vi "seat leak test.vi"(7 "LabVIEW Web Service Request":refnum<class "Web Request.lvclass">, 10 "testPressure":dbl, 11 "time":dbl) -> ()   [LabVIEW 2015]
uses:
  <vilib>/wsapi/Web Request.lvclass
  <vilib>/Waveform/WDTOps.llb/WDT Append Waveforms DBL.vi
panel:
  out "value":string
  in  "Start timer":bool
  out "Final Pressure":dbl
  out "data":waveform(dbl)[](graph)
  out "timer":dbl
  in  "Stop timer":bool
  in  "Stop (Pressure Reading)":bool
  out "Starting Pressure":dbl format="%#_2g"
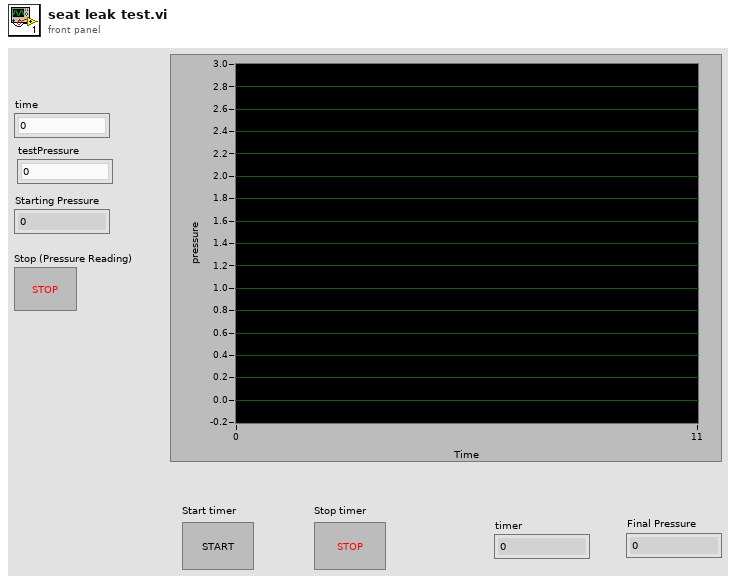
[diagram p1: front panel]
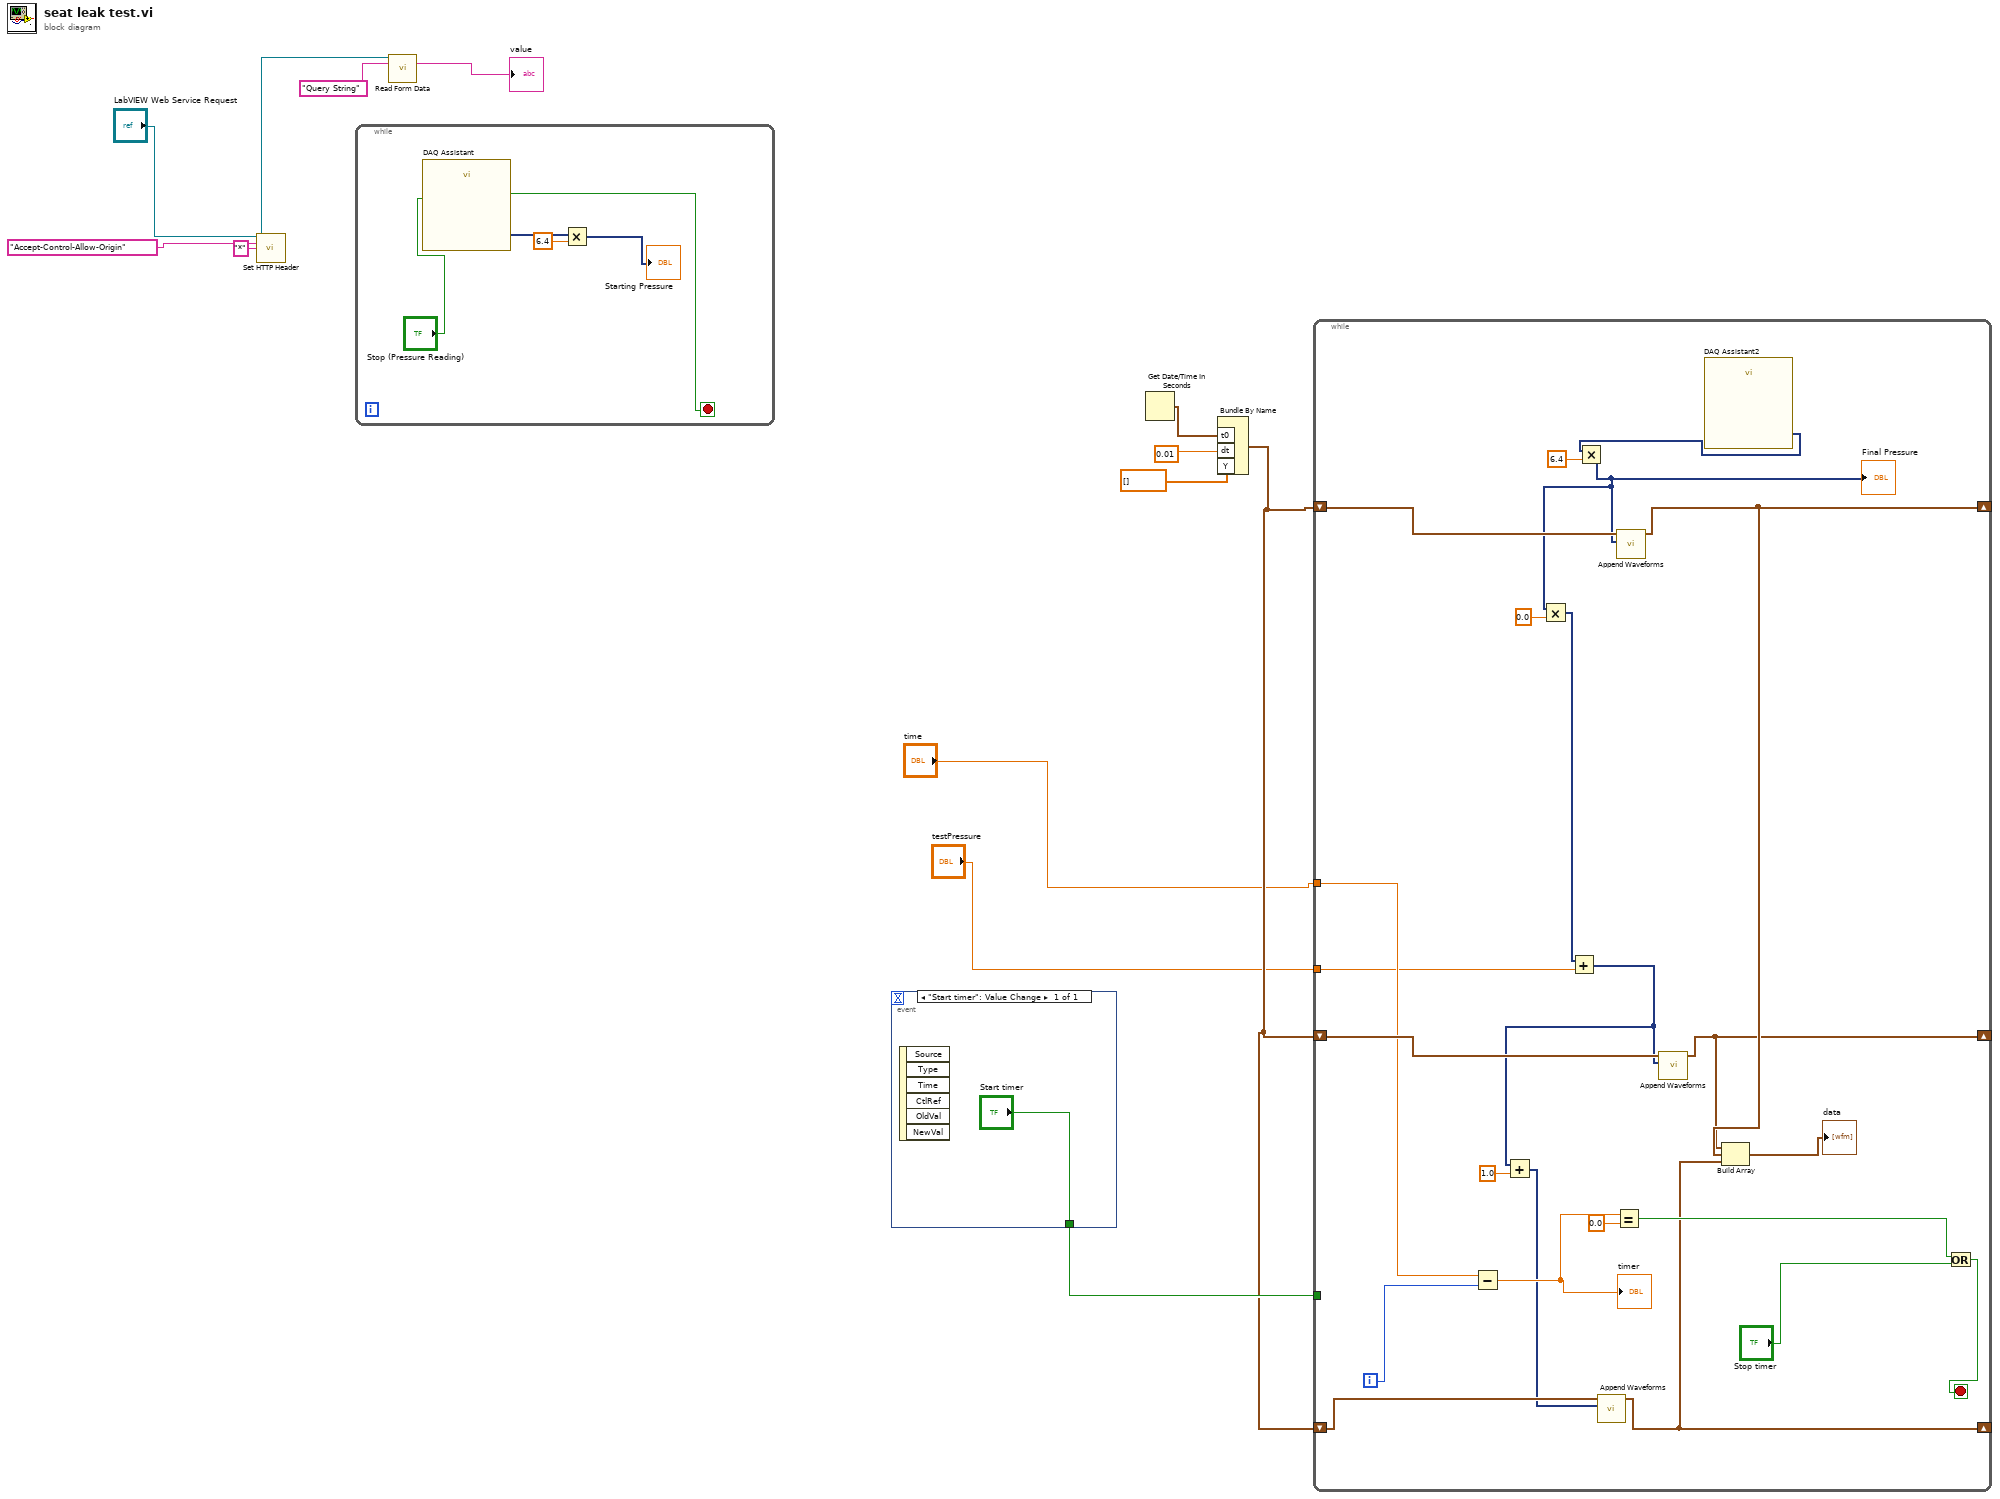
[diagram p0: block diagram]
diagram:
  n1 = call <vilib>:"Set HTTP Header.vi"("LabVIEW Web Service Request"="LabVIEW Web Service Request", "header"="Accept-Control-Allow-Origin", "header value"="*") -> ("LabVIEW Web Service Request out"=w5:refnum<class "Web Request.lvclass">)  [unwired: 11 in, 1 out]
  n2 = while {
    stop <- w14 stop-if-true
    n3 = call "DAQ Assistant"("stop (F)"="Stop (Pressure Reading)") -> ("data"=w18:dynamicdata, "stopped"=w14:bool)  [unwired: 15 in, 2 out]
    n4 = Multiply(x=w18, y=6.4) -> (x*y=→"Starting Pressure":dynamicdata)
  }
  n5 = call <vilib>:"Read Form Data.vi"("LabVIEW Web Service Request"=w5, "key"="Query String") -> ("value"=→"value":string)  [unwired: 10 in, 3 out]
  n6 = event shown="[0] \"Start timer\": Value Change" {
    selector: _ -> [_]
    dyn-events: _ -> [_]
    timeout: _ -> [_]
    tunnel: ["Start timer"] -> w10
    event "Start timer": Value Change {
      n7 = event-data() -> ()  [unwired: 1 in, 6 out]
    }
  }
  n8 = Get Date/Time In Seconds() -> (seconds since 1Jan1904=w13:timestamp)
  n9 = Bundle By Name("t0"=w13, "dt"=0.01, "Y"=dbl[] []) -> (w9:waveform(dbl))  [unwired: 1 in]
  n10 = while {
    shift-right: [w36] -> _
    shift-left: w9 -> [w42]
    tunnel: "time" -> [w30]
    shift-right: [w35] -> _
    shift-left: w9 -> [w40]
    tunnel: w10 -> [_]
    shift-right: [w21] -> _
    shift-left: w9 -> [w25]
    tunnel: "testPressure" -> [w20]
    i -> [w31]
    stop <- w33 stop-if-true
    n11 = Subtract(x=w30, y=w31) -> (x-y=w29:dbl)
    "timer" <- w29
    n12 = Equal?(x=w29, y=0.0) -> (x = y?=w27:bool)
    n13 = call "DAQ Assistant2"() -> ("data"=w34:dynamicdata)  [unwired: 16 in, 3 out]
    n14 = Multiply(x=w34, y=6.4) -> (x*y=w39:dynamicdata)
    "Final Pressure" <- w39
    n15 = Multiply(x=w39, y=0.0) -> (x*y=w37:dynamicdata)
    n16 = Add(x=w37, y=w20) -> (x+y=w24:dynamicdata)
    n17 = Add(x=w24, y=1.0) -> (x+y=w22:dynamicdata)
    n18 = call-poly <vilib>:"Append Waveforms.vi"("waveform B"=w22, "waveform A"=w25) -> ("waveform out"=w21:waveform(dbl))  [unwired: 8 in, 1 out]
    n19 = call-poly <vilib>:"Append Waveforms.vi"("waveform B"=w39, "waveform A"=w42) -> ("waveform out"=w36:waveform(dbl))  [unwired: 8 in, 1 out]
    n20 = call-poly <vilib>:"Append Waveforms.vi"("waveform B"=w24, "waveform A"=w40) -> ("waveform out"=w35:waveform(dbl))  [unwired: 8 in, 1 out]
    n21 = Build Array(w35, w36, w21) -> (→"data":waveform(dbl)[])
    n22 = Or(x=w27, y="Stop timer") -> (x .or. y?=w33:bool)
  }
